vi "Diode-Control-Panel.vi"() -> ()   [LabVIEW 2020]
panel:
  in  "Previous Button":bool
  in  "Next Button":bool
  out "Keyword Info":T1
  in  "Stop Program":bool
  in  "Open Device":bool
  in  "Close Device":bool
  in  "IP Address of Device":string="192.168.203.151"
  out "Return Value":string
  in  "Set Value":string
  in  "Set":bool
  in  "Get":bool
  # "(Close device first)"
  # "Buttons become usable after opening device"
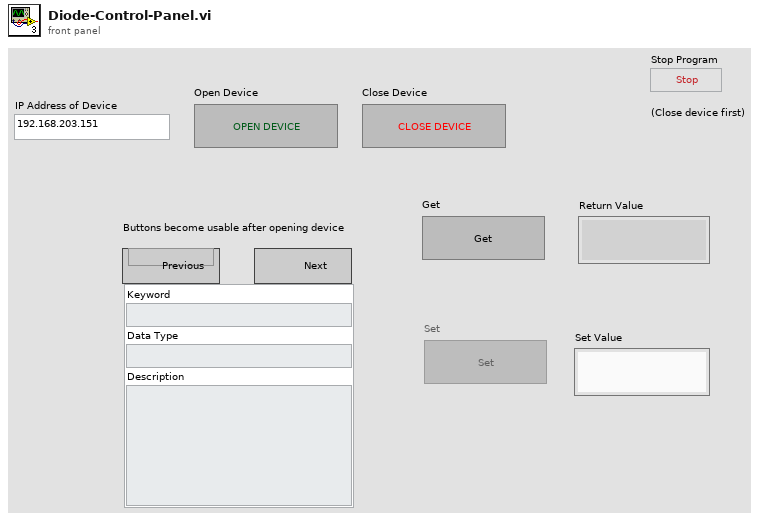
[diagram p1: front panel]
types:
  T1 = cluster{"Keyword":string, "Data Type":string, "Description":string}
  T2 = enum8{"Enabled", "Disabled", "Disabled and Grayed Out"}
  T3 = typedef "Diode-Keyword.ctl" = cluster{"Keyword":string, "Gettable":bool, "Settable":bool, "Is Array":bool, "Data Type":string, "Description":string}
  T4 = cluster{"Keyword":string, "Is Array":bool, "Data Type":string}
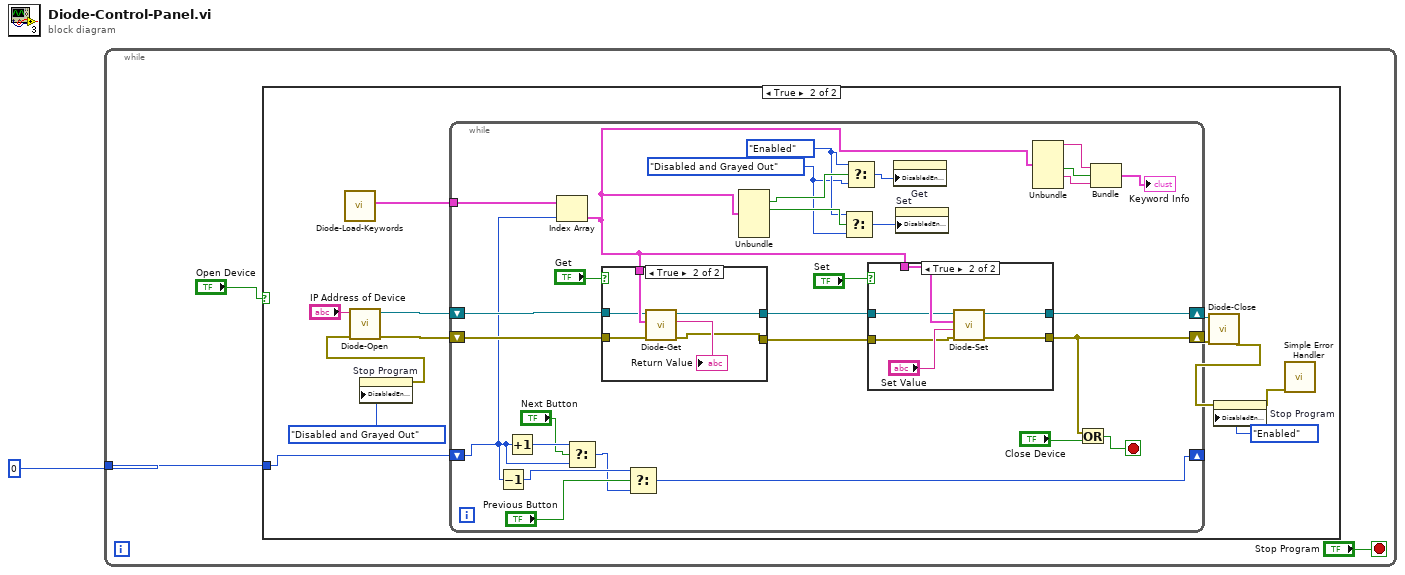
[diagram p0: block diagram]
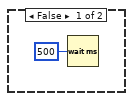
[diagram p2: hidden frame]
diagram:
  n1 = while {
    tunnel: 0 ("Keyword Selection 2") -> [w2]
    stop <- "Stop Program" stop-if-true
    n2 = case shown="True" "Open Device" {
      tunnel: w2 -> [_ w6]
      frame False {
        n3 = Wait (ms)(milliseconds to wait=u32 500) -> ()  [unwired: 1 out]
      }
      frame True {
        n4 = call "Diode-Load-Keywords.vi"() -> ("Diodes Keywords Array"=w17:T3[])  [unwired: 11 in]
        n5 = property on="Stop Program" class="Bool"("DisabledEnum"=T2."Disabled and Grayed Out" ("Disabled")) -> (error out=w8:errorcluster)  [unwired: 2 in, 1 out]
        n6 = call "Diode-Open.vi"("error in (no error)"=w8, "IP Address of Diode"="IP Address of Device") -> ("error out"=w9:errorcluster, "connection ID"=w15:refnum<k5>)  [unwired: 8 in]
        n7 = while {
          tunnel: w17 -> [w46]
          shift-right: [w36] -> w12
          shift-left: w9 -> [w41]
          shift-right: [w40] -> w16
          shift-left: w15 -> [w39]
          shift-right: [w20] -> _
          shift-left: w6 -> [w19]
          stop <- w38 stop-if-true
          w31 = T2."Disabled and Grayed Out" ("Disabled")
          w32 = T2."Enabled" ("Disabled")
          n8 = Decrement(x=w19) -> (x-1=w24:i32)
          n9 = Increment(x=w19) -> (x+1=w25:i32)
          n10 = Index Array(array=w46, index=w19) -> (element=w18:T3)
          n11 = Select(t=w25, s="Next Button", f=w19) -> (s? t:f=w21:i32)
          n12 = case shown="True" "Get" {
            tunnel: w18 -> [_ w61]
            tunnel: [w55 w60] -> w43
            tunnel: [w56 w59] -> w42
            tunnel: w41 -> [w56 w58]
            tunnel: w39 -> [w55 w57]
            frame False {
            }
            frame True {
              n13 = call "Diode-Get.vi"("error in (no error)"=w58, "Diode Keyword"=w61, "connection ID"=w57) -> ("error out"=w59:errorcluster, "Response"=→"Return Value":string, "connection ID out"=w60:refnum<k5>)  [unwired: 6 in]
            }
          }
          n14 = Select(t=w24, s="Previous Button", f=w21) -> (s? t:f=w20:i32)
          n15 = Unbundle(w18) -> ("Gettable"=w35:bool, "Settable"=w33:bool)  [unwired: 4 out]
          n16 = Select(t=w32, s=w33, f=w31) -> (s? t:f=w34:T2)
          n17 = Select(t=w32, s=w35, f=w31) -> (s? t:f=w30:T2)
          n18 = case shown="True" "Set" {
            tunnel: w18 -> [_ w53]
            tunnel: w43 -> [w47 w52]
            tunnel: [w47 w51] -> w40
            tunnel: [w48 w50] -> w36
            tunnel: w42 -> [w48 w49]
            frame False {
            }
            frame True {
              n19 = call "Diode-Set.vi"("error in (no error)"=w49, "Set Value"="Set Value", "Diode Keyword"=w53, "connection ID"=w52) -> ("error out"=w50:errorcluster, "connection ID out"=w51:refnum<k5>)  [unwired: 6 in]
            }
          }
          n20 = property on="Get" class="Bool"("DisabledEnum"=w30) -> ()  [unwired: 2 in, 2 out]
          n21 = property on="Set" class="Bool"("DisabledEnum"=w34) -> ()  [unwired: 2 in, 2 out]
          n22 = Unbundle(w18) -> ("Keyword"=w29:string, "Is Array"=w28:bool, "Data Type"=w27:string)  [unwired: 3 out]
          n23 = Or(x=w36, y="Close Device") -> (x .or. y?=w38:bool)
          n24 = Bundle("Keyword"=w29, "Is Array"=w28, "Data Type"=w27) -> (→"Keyword Info":T4)  [unwired: 1 in]
        }
        n25 = call "Diode-Close.vi"("error in (no error)"=w12, "connection ID"=w16) -> ("error out"=w11:errorcluster)  [unwired: 9 in]
        n26 = property on="Stop Program" class="Bool"(error in=w11, "DisabledEnum"=T2."Enabled" ("Disabled")) -> (error out=w7:errorcluster)  [unwired: 1 in, 1 out]
        n27 = call <vilib>:"Simple Error Handler.vi"("error in (no error)"=w7) -> ()  [unwired: 4 in, 5 out]
      }
    }
  }
